vi "Lex Symbol.vi"(8 "error in (no error)":errorcluster, 11 "JSON Lexer in":refnum<class "JSON Lexer.lvclass">) -> (0 "error out":errorcluster, 1 "EOF":bool, 2 "Next State":T1=enum."Value", 3 "JSON Lexer out":refnum<class "JSON Lexer.lvclass">)   [LabVIEW 2019, in "JKI JSON Serialization.lvlib" / "JSON Lexer.lvclass"]
doc: "JKI JSON 1.1.10.37\nTomi Maila - JKI\nCopyright (c) 2017, JKI"
uses:
  JSON Lexer.lvclass
  JSON Lexer States.ctl
  JSON Token Type.ctl
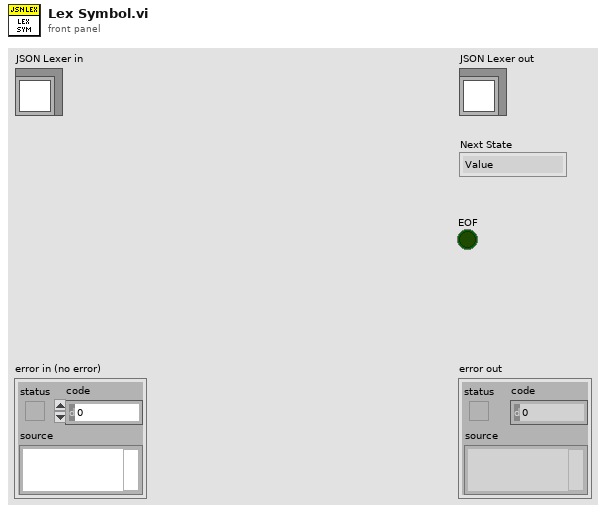
[diagram p1: front panel]
types:
  T1 = typedef "JKI JSON Serialization.lvlib/JSON Lexer.lvclass/JSON Lexer States.ctl" = enum16{"Undefined", "Value", "String", "Numeric", "Number", "Symbol", "Symbolic Number"}
  T2 = typedef "JKI JSON Serialization.lvlib/JSON Lexer.lvclass/JSON Token Type.ctl" = enum32{"unknown", "comma", "end-label", "begin-object", "end-object", "begin-array", "end-array", "quoted-string", "boolean", "exponential-number", "decimal-number", "integer-number", "special-number", "null", "symbol", "whitespace", "EOF"}
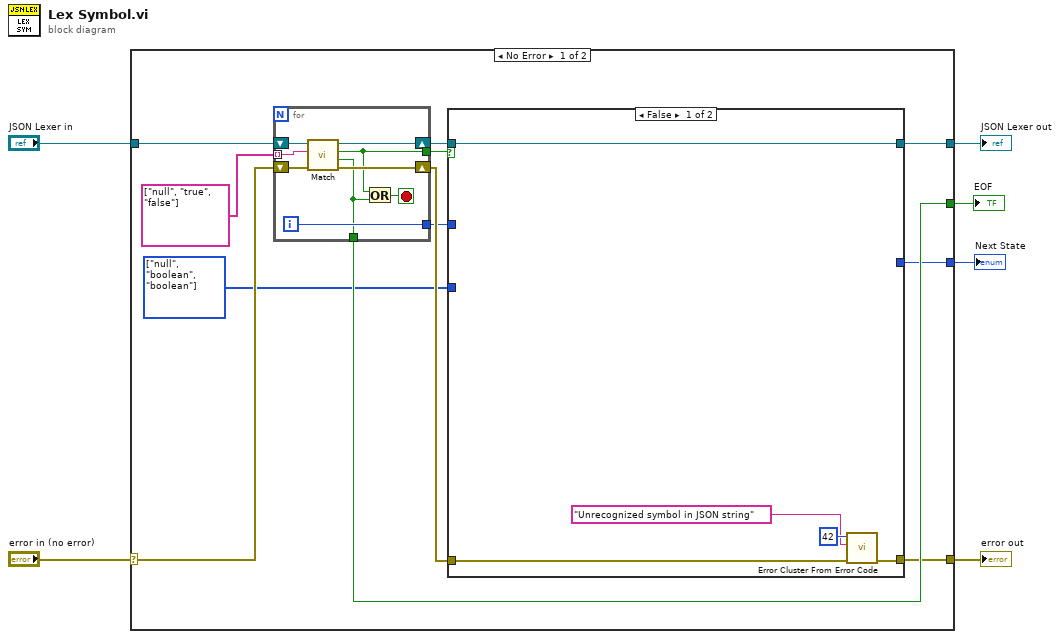
[diagram p0: block diagram]
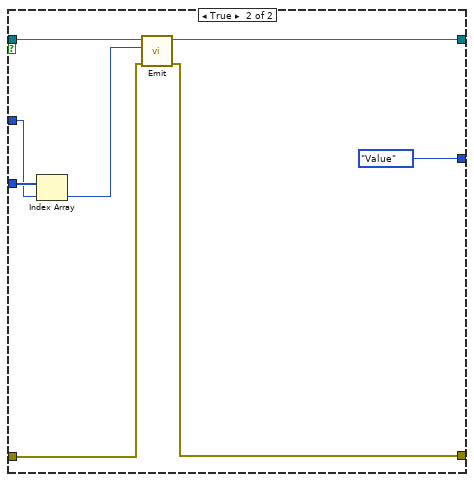
[diagram p2: hidden frame]
diagram:
  n1 = case shown="No Error" "error in (no error)" {
    selector: "error in (no error)" -> [w17 w42]
    tunnel: [w12 w42] -> w5
    tunnel: [w8 w41] -> w3
    tunnel: "JSON Lexer in" -> [w18 w41]
    tunnel: [w14 _] -> w2
    tunnel: [w7 _] -> w1
    frame No Error {
      w11 = T2[] [enum."null", enum."boolean", enum."boolean"] items=["unknown", "comma", "end-label", "begin-object", "end-object", "begin-array", "end-array", "quoted-string", "boolean", "exponential-number", "decimal-number", "integer-number", "special-number", "null", "symbol", "whitespace", "EOF"]
      n2 = for {
        shift-right: [w39] -> w10
        shift-left: w18 -> [w40]
        shift-right: [w36] -> w13
        shift-left: w17 -> [w37]
        tunnel: string[] ["null", "true", "false"] -> [w35] mode=indexing
        tunnel: [w34] -> w9
        tunnel: [w33] -> w15
        tunnel: [w32] -> w14
        i -> [w34]
        stop <- w38 stop-if-true
        n3 = call "Match.vi"("error in (no error)"=w37, "Match String"=w35, "JSON Lexer in"=w40) -> ("error out"=w36:errorcluster, "EOF"=w32:bool, "Matched?"=w33:bool, "JSON Lexer out"=w39:refnum<class "JSON Lexer.lvclass">)  [unwired: 5 in]
        n4 = Or(x=w33, y=w32) -> (x .or. y?=w38:bool)
      }
      n5 = case shown="False" w15 {
        tunnel: w13 -> [w21 w27]
        tunnel: [w22 w26] -> w12
        tunnel: w11 -> [_ w31]
        tunnel: w10 -> [w23 w29]
        tunnel: w9 -> [_ w30]
        tunnel: [w23 w28] -> w8
        tunnel: [_ JSON_Lexer_States."Value" ("JSON Lexer State")] -> w7
        frame False {
          n6 = call <vilib>:"Error Cluster From Error Code.vi"("error in (no error)"=w21, "error message (\"\")"="Unrecognized symbol in JSON string", "error code (0)"=42) -> ("error out"=w22:errorcluster)  [unwired: 6 in]
        }
        frame True {
          n7 = Index Array(array=w31, index=w30) -> (element=w25:T2)
          n8 = call "Emit.vi"("error in (no error)"=w27, "JSON Token Type"=w25, "JSON Lexer in"=w29) -> ("error out"=w26:errorcluster, "JSON Lexer out"=w28:refnum<class "JSON Lexer.lvclass">)  [unwired: 7 in]
        }
      }
    }
    frame Error {
    }
  }
  "error out" <- w5
  "JSON Lexer out" <- w3
  "Next State" <- w1
  "EOF" <- w2
